vi "Ballard XML Generator.Add SSM Channel.vi"(10 "create SSM chan?":bool, 11 "string in":string) -> (3 "string out":string)   [LabVIEW 2020]
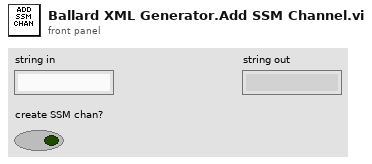
[diagram p1: front panel]
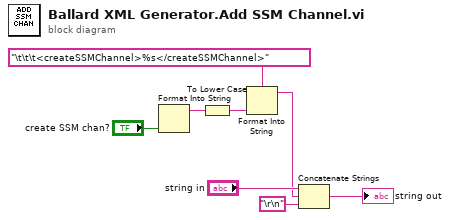
[diagram p0: block diagram]
diagram:
  n1 = Format Into String("create SSM chan?") -> (resulting string=w2:string)  [unwired: 3 in, 1 out]
  n2 = To Lower Case(string=w2) -> (all lower case string=w1:string)
  n3 = Format Into String(format string="\t\t\t<createSSMChannel>%s</createSSMChannel>", w1) -> (resulting string=w4:string)  [unwired: 2 in, 1 out]
  n4 = Concatenate Strings("string in", w4, "\r\n") -> (→"string out":string)
